vi "Formula_node_ejercicio.vi"() -> ()   [LabVIEW 2020]
panel:
  out "XY Graph":cluster{dbl[], dbl[]}(graph)
  out "Waveform Graph":dbl[](graph)
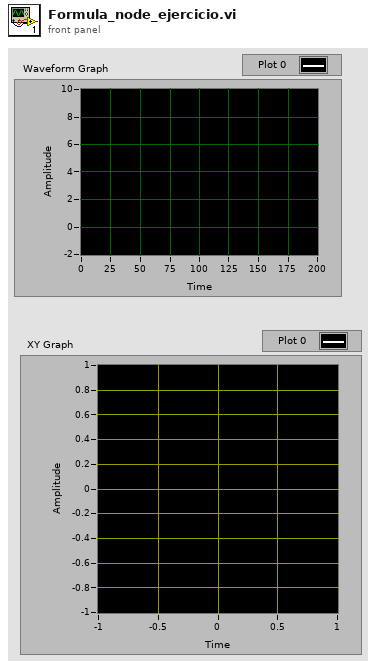
[diagram p1: front panel]
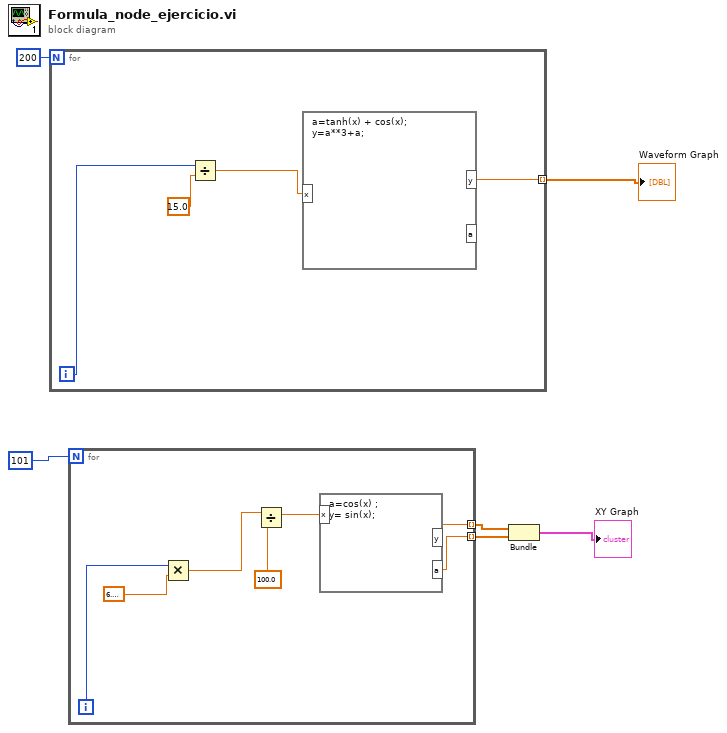
[diagram p0: block diagram]
diagram:
  n1 = for {
    N: 200 -> [_]
    tunnel: [w7] -> w6 mode=indexing
    i -> [w9]
    n2 = Divide(x=w9, y=15.0) -> (x/y=w8:dbl)
    n3 = formula code="a=tanh(x) + cos(x);\ny=a**3+a;"("x"=w8) -> ("y"=w7:dbl)  [unwired: 1 out]
  }
  "Waveform Graph" <- w6
  n4 = for {
    N: 101 -> [_]
    tunnel: [w12] -> w3 mode=indexing
    tunnel: [w11] -> w2 mode=indexing
    i -> [w16]
    n5 = Multiply(x=w16, y=6.283185307179586) -> (x*y=w15:dbl)
    n6 = Divide(x=w15, y=100.0) -> (x/y=w13:dbl)
    n7 = formula code="a=cos(x) ;\ny= sin(x);"("x"=w13) -> ("y"=w12:dbl, "a"=w11:dbl)
  }
  n8 = Bundle(w3, w2) -> (→"XY Graph":cluster{dbl[], dbl[]})  [unwired: 1 in]
